vi "Log FFT.vi"   [LabVIEW 2012]
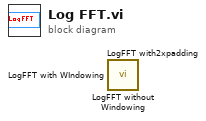
[diagram p0: block diagram]
diagram:
  n1 = call <userlib>:"LogFFT without Windowing.vi"() -> ()  [unwired: 11 in, 1 out]
  n2 = call <userlib>:"LogFFT with2xpadding.vi"() -> ()  [unwired: 11 in, 1 out]
  n3 = call <userlib>:"LogFFT with WIndowing.vi"() -> ()  [unwired: 11 in, 1 out]
